vi "Download_LatexPackages_GetZipFile.vi"(10 "Save Path - Folder":path=path "C:/Temp/Latex/Packages", 11 "package list (In)":string[](array[string])) -> ()   [LabVIEW 2014]
uses:
  <vilib>/httpClient/LabVIEWHTTPClient.lvlib
  <vilib>/zip/NI_Unzip.lvlib
panel:
  in  "Error In":errorcluster
  out "Error from unzipping":errorcluster[](array[cluster])
  out "error out":errorcluster
  out "bodies":string[](array[string])
  out "headers":string[](array[string])
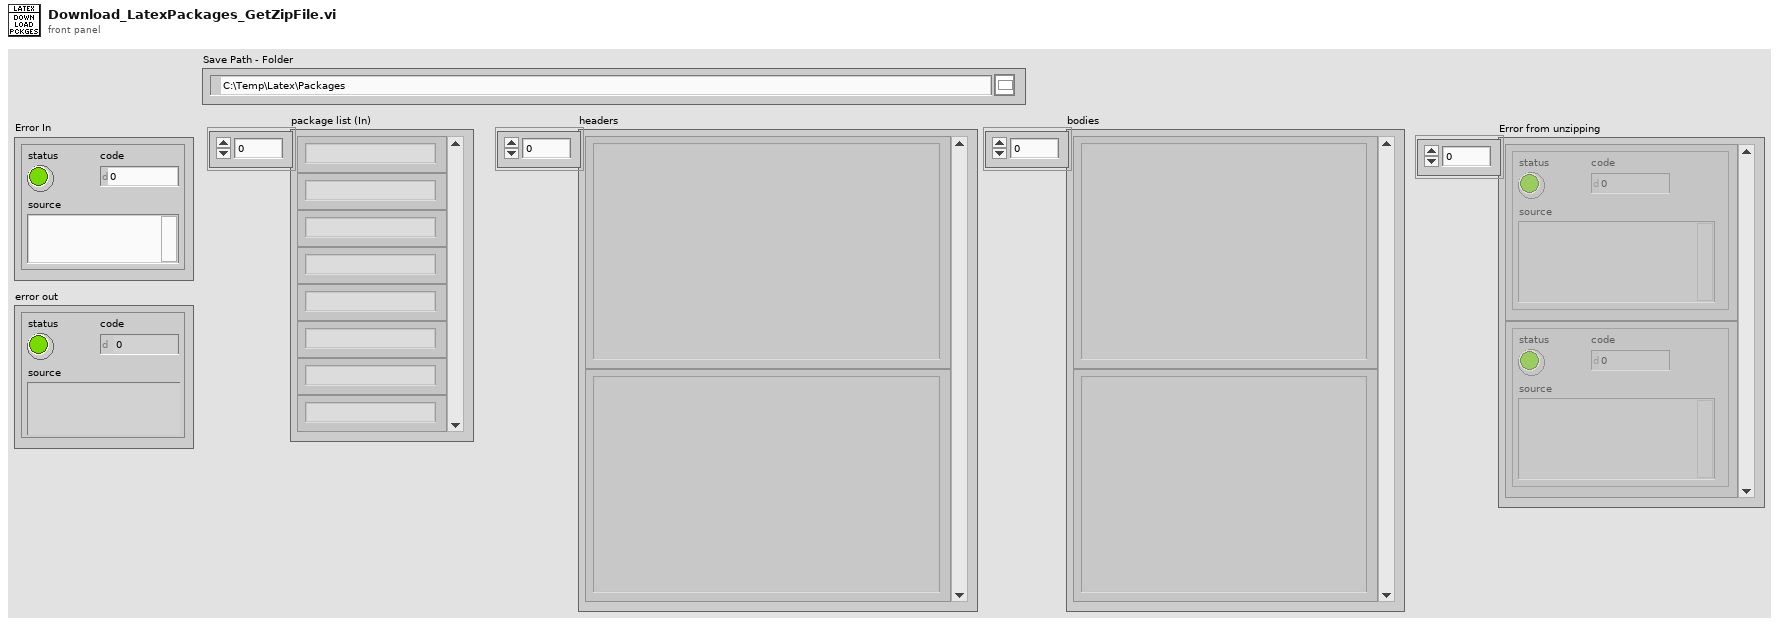
[diagram p1: front panel]
types:
  T1 = typedef "LabVIEWHTTPClient.lvlib/ClientHandle.ctl" = refnum<k1>
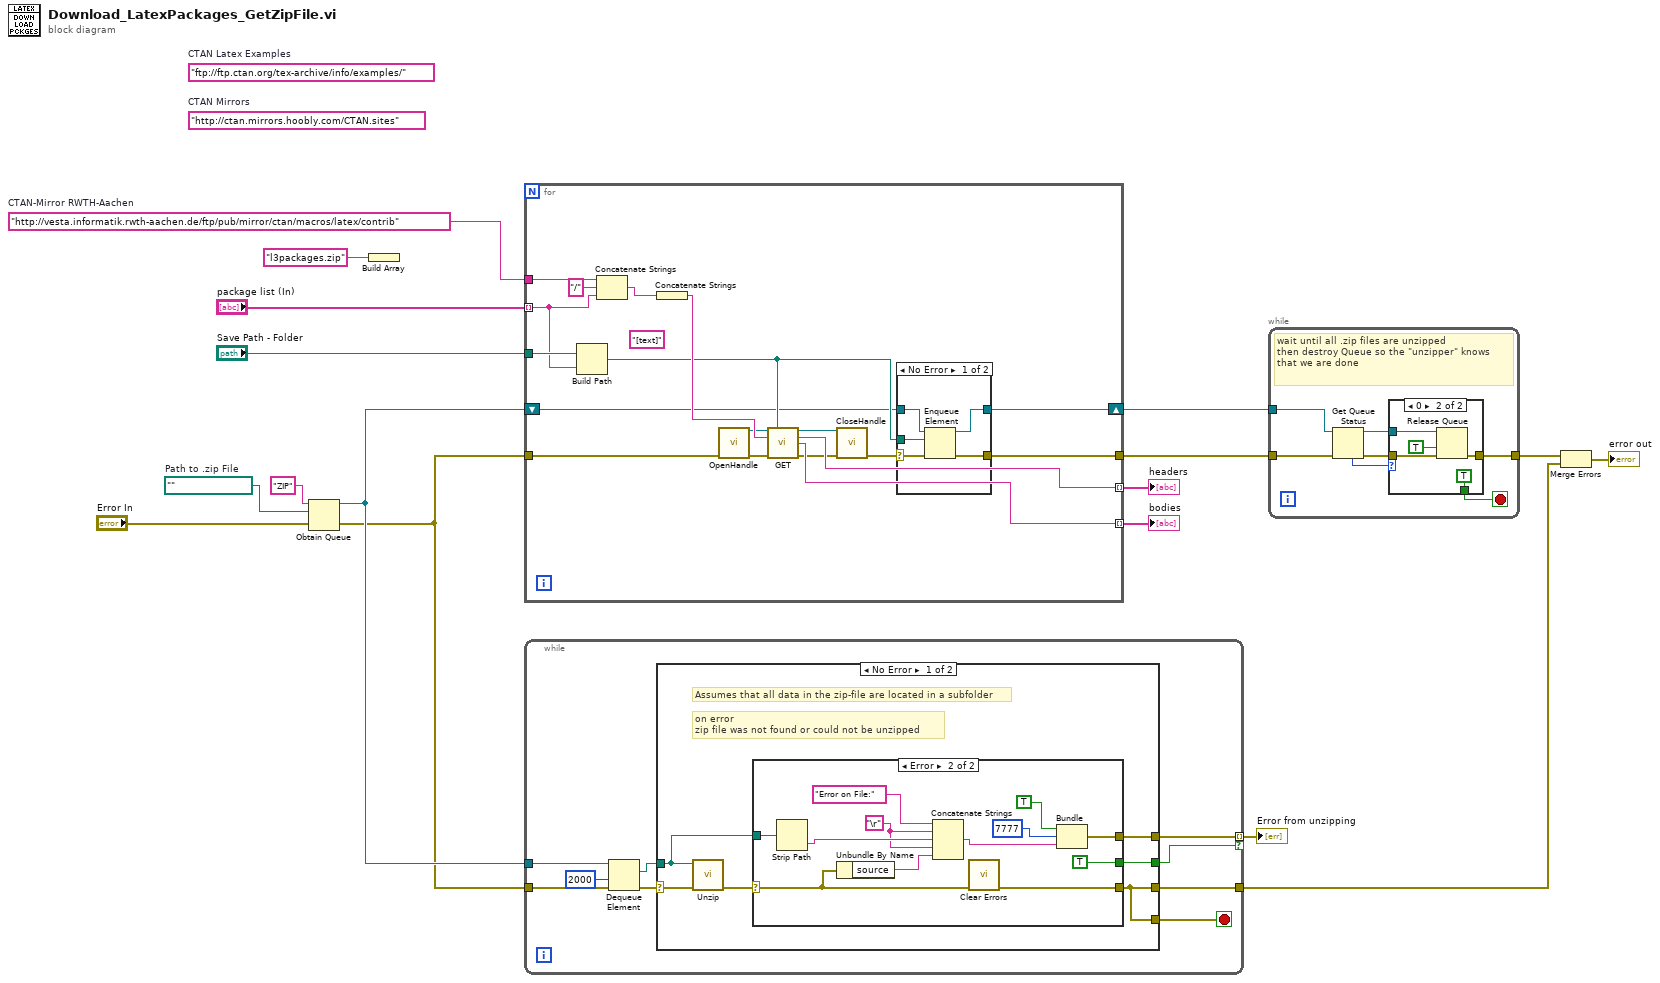
[diagram p0: block diagram]
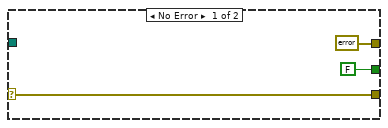
[diagram p3: hidden frame]
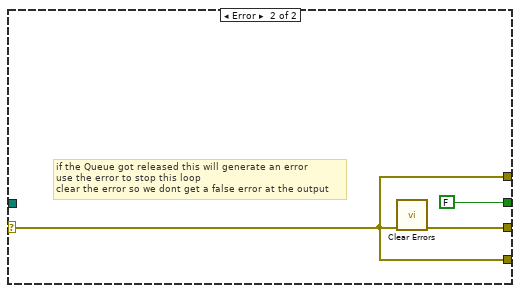
[diagram p4: hidden frame]
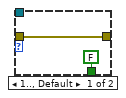
[diagram p5: hidden frame]
diagram:
  (unwired) "http://ctan.mirrors.hoobly.com/CTAN.sites"  # CTAN Mirrors
  (unwired) "ftp://ftp.ctan.org/tex-archive/info/examples/"  # CTAN Latex Examples
  w11 = path ""  # Path to .zip File
  w12 = "http://vesta.informatik.rwth-aachen.de/ftp/pub/mirror/ctan/macros/latex/contrib"  # CTAN-Mirror RWTH-Aachen
  n1 = Obtain Queue(name (unnamed)="ZIP", element data type=w11) -> (queue out=w9:refnum<queue>)  [unwired: 3 in, 2 out]
  n2 = Build Array("l3packages.zip" ("string")) -> ()  [unwired: 1 out]
  n3 = for {
    tunnel: w12 -> [w30]
    tunnel: "package list (In)" -> [w28] mode=indexing
    tunnel: "Save Path - Folder" -> [w34]
    tunnel: [w31] -> w7
    tunnel: [w26] -> w13 mode=indexing
    tunnel: [w25] -> w14 mode=indexing
    tunnel: "Error In" -> [w17]
    shift-right: [w23] -> w6
    shift-left: w9 -> [w24]
    (unwired) "[text]" ("string")
    n4 = Build Path(base path=w34, name or relative path=w28) -> (appended path=w32:path)
    n5 = Concatenate Strings(w30, "/" ("string"), w28) -> (w29:string)
    n6 = Concatenate Strings(w29) -> (w33:string)
    n7 = call <vilib>:"OpenHandle.vi"("error in (no error)"=w17) -> ("client handle out"=w19:T1, "error out"=w21:errorcluster)  [unwired: 13 in]
    n8 = call <vilib>:"GET.vi"("client handle"=w19, "output file"=w32, "url"=w33, "error in (no error)"=w21) -> ("client handle out"=w20:T1, "headers"=w25:string, "body"=w26:string, "error out"=w22:errorcluster)  [unwired: 8 in]
    n9 = call <vilib>:"CloseHandle.vi"("client handle"=w20, "error in (no error)"=w22) -> ("error out"=w18:errorcluster)  [unwired: 13 in]
    n10 = case shown="No Error" w18 {
      selector: w18 -> [w38 w41]
      tunnel: [w39 w41] -> w31
      tunnel: w32 -> [w37 _]
      tunnel: w24 -> [w36 w40]
      tunnel: [w35 w40] -> w23
      frame No Error {
        n11 = Enqueue Element(queue=w36, element=w37, error in (no error)=w38) -> (queue out=w35:refnum<queue>, error out=w39:errorcluster)  [unwired: 1 in, 1 out]
      }
      frame Error {
      }
    }
  }
  "headers" <- w14
  "bodies" <- w13
  n12 = while {
    tunnel: w9 -> [w50]
    tunnel: [w47] -> w4
    tunnel: [w44] -> w3 mode=indexing if=w43
    tunnel: "Error In" -> [w42]
    stop <- w45 stop-if-true
    n13 = Dequeue Element(queue=w50, timeout in ms (-1)=2000, error in (no error)=w42) -> (element=w49:path, error out=w48:errorcluster)  [unwired: 2 out]
    n14 = case shown="No Error" w48 {
      selector: w48 -> [w56 w72]
      tunnel: w49 -> [w53 _]
      tunnel: [w55 w74] -> w47
      tunnel: [w55 w72] -> w45
      tunnel: [w54 w72] -> w44
      tunnel: [w51 FALSE] -> w43
      frame No Error {
        # "Assumes that all data in the zip-file are located in a subfolder"
        # "on error\nzip file was not found or could not be unzipped"
        n15 = call <vilib>:"Unzip.vi"("error in (no error)"=w56, "Zip file"=w53) -> ("error out"=w52:errorcluster)  [unwired: 7 in, 2 out]
        n16 = case shown="Error" w52 {
          selector: w52 -> [w59 w62]
          tunnel: [w59 w71] -> w55
          tunnel: [errorcluster {FALSE, 0, ""} w70] -> w54
          tunnel: w53 -> [_ w67]
          tunnel: [FALSE TRUE] -> w51
          frame No Error {
          }
          frame Error {
            w60 = "\r"
            n17 = Strip Path(path=w67) -> (name=w66:string)  [unwired: 1 out]
            n18 = Unbundle By Name(w62) -> ("source"=w68:string)
            n19 = Concatenate Strings("Error on File:" ("string"), w60, w66, w60, w68) -> (w64:string)
            n20 = call <vilib>:"Clear Errors.vi"("error in (no error)"=w62) -> ("error out"=w71:errorcluster)  [unwired: 5 in, 1 out]
            n21 = Bundle(TRUE, 7777, w64) -> (w70:errorcluster)  [unwired: 1 in]
          }
        }
      }
      frame Error {
        # "if the Queue got released this will generate an error\nuse the error to stop this loop\nclear the error so we dont get a false error at the output"
        n22 = call <vilib>:"Clear Errors.vi"("error in (no error)"=w72) -> ("error out"=w74:errorcluster)  [unwired: 5 in, 1 out]
      }
    }
  }
  "Error from unzipping" <- w3
  n23 = while {
    tunnel: [w81] -> w8
    tunnel: w7 -> [w80]
    tunnel: w6 -> [w76]
    stop <- w75 stop-if-true
    # "wait until all .zip files are unzipped\nthen destroy Queue so the \"unzipper\" knows that we are done"
    n24 = Get Queue Status(queue=w76, error in (no error)=w80) -> (queue out=w77:refnum<queue>, error out=w79:errorcluster, # elements in queue=w78:i32)  [unwired: 1 in, 5 out]
    n25 = case shown="0" w78 {
      tunnel: [w83 w88] -> w81
      tunnel: w79 -> [w83 w87]
      tunnel: w77 -> [_ w86]
      tunnel: [FALSE TRUE] -> w75
      frame 1.., Default {
      }
      frame 0 {
        n26 = Release Queue(queue=w86, force destroy? (F)=TRUE, error in (no error)=w87) -> (error out=w88:errorcluster)  [unwired: 2 out]
      }
    }
  }
  n27 = Merge Errors(w8, w4) -> (→"error out":errorcluster)
